vi "Get Scope Timebase Values.vi"(2 "error in (no error)":errorcluster) -> (0 "error out":errorcluster, 1 "Timebase Values Array":dbl[](array[numeric]))   [LabVIEW 2020]
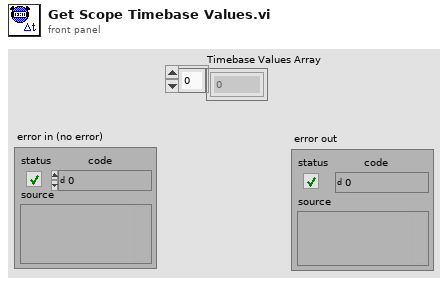
[diagram p1: front panel]
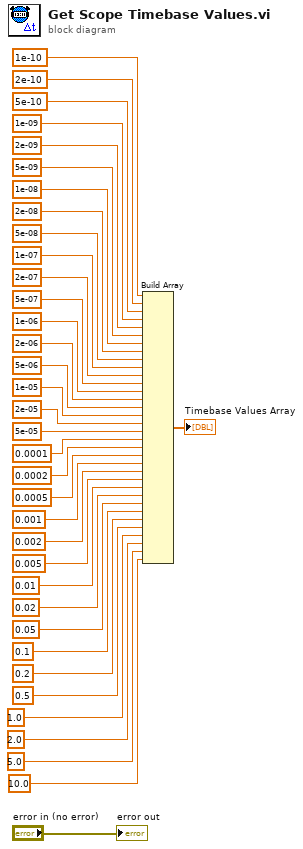
[diagram p0: block diagram]
diagram:
  n1 = Build Array(1e-10, 2e-10, 5e-10, 1e-09, 2e-09, 5e-09, 1e-08, 2e-08, 5e-08, 1e-07, 2e-07, 5e-07, 1e-06, 2e-06, 5e-06, 1e-05, 2e-05, 5e-05, 0.0001, 0.0002, 0.0005, 0.001, 0.002, 0.005, 0.01, 0.02, 0.05, 0.1, 0.2, 0.5, 1.0, 2.0, 5.0, 10.0) -> (→"Timebase Values Array":dbl[])
  "error out" <- "error in (no error)"
